vi "IMU_Logger_simple.vi"() -> ()   [LabVIEW 2013]
uses:
  IMU_Data_Type_Def.ctl
  <vilib>/Utility/file.llb/Write To Spreadsheet File (DBL).vi
panel:
  out "Less then 100Hz":bool
  out "IMU_Data_simple":T1
  out "Elapsed Time":u32
  in  "Stop Button":bool
  out "error out":errorcluster
  out "Filename Out":path
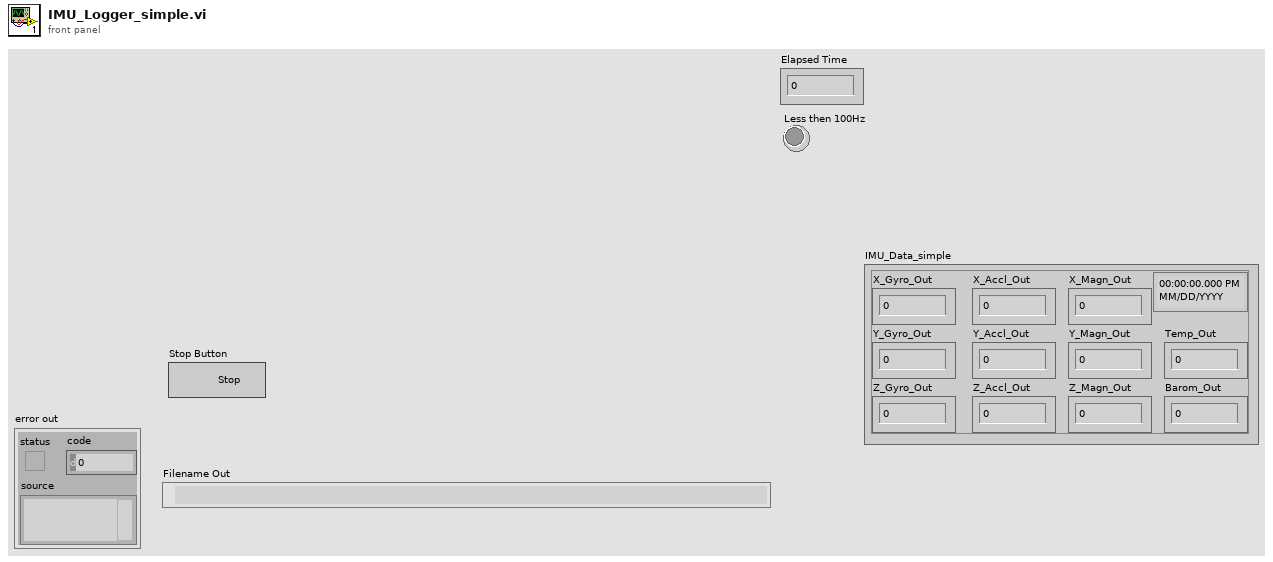
[diagram p1: front panel]
types:
  T1 = typedef "IMU_Data_Type_Def.ctl" = cluster{timestamp, "X_Gyro_Out":dbl, "Y_Gyro_Out":dbl, "Z_Gyro_Out":dbl, "X_Accl_Out":dbl, "Y_Accl_Out":dbl, "Z_Accl_Out":dbl, "X_Magn_Out":dbl, "Y_Magn_Out":dbl, "Z_Magn_Out":dbl, "Temp_Out":dbl, "Barom_Out":dbl}
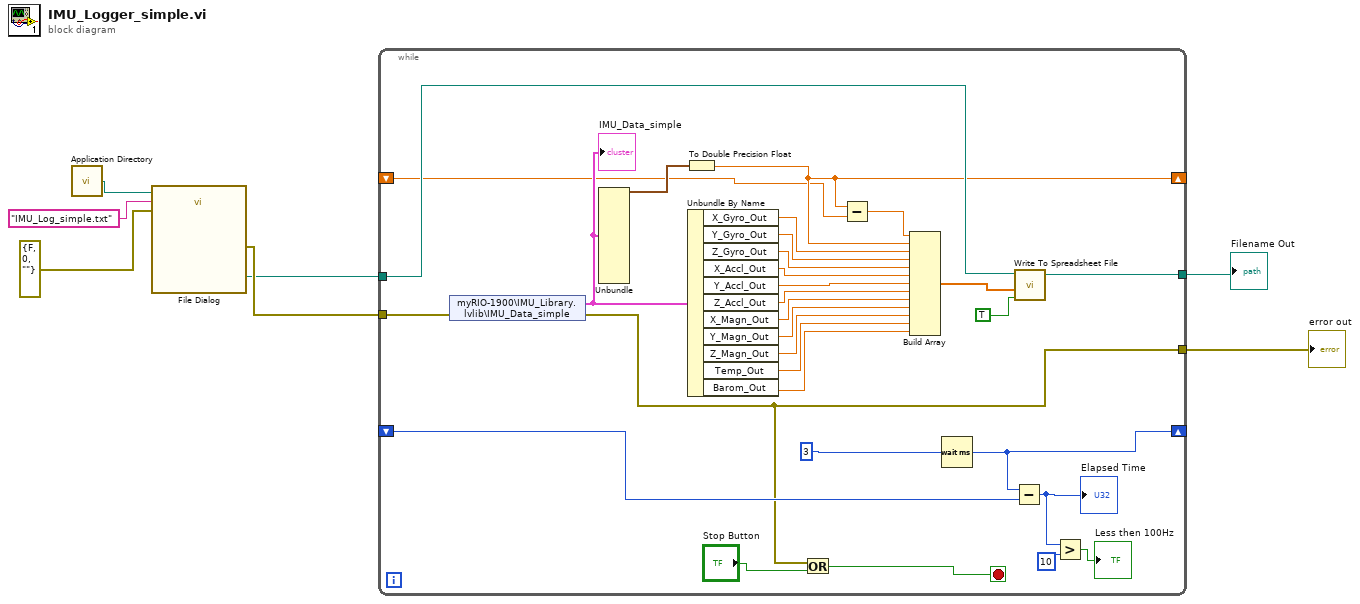
[diagram p0: block diagram]
diagram:
  n1 = call <vilib>:"Application Directory.vi"() -> ("Application Directory"=w7:path)
  n2 = call "File Dialog"("start path"=w7, "default name"="IMU_Log_simple.txt" ("name or relative path"), "error in"=errorcluster {"status"=FALSE, "code"=0, "source"=""} ("error in (no error)")) -> ("selected path"=w2:path, "error out"=w4:errorcluster)  [unwired: 9 in, 2 out]
  n3 = while {
    shift-right: [w15] -> _
    shift-left: _ -> [w35]
    tunnel: w4 -> [w19]
    tunnel: [w18] -> w3
    tunnel: w2 -> [w17]
    tunnel: [w16] -> w1
    shift-right: [w9] -> _
    shift-left: _ -> [w8]
    stop <- w24 stop-if-true
    n4 = shared-variable "myRIO-1900\\IMU_Library.lvlib\\IMU_Data_simple"(error in=w19) -> (w21:T1, error out=w18:errorcluster)
    "IMU_Data_simple" <- w21
    n5 = Unbundle(w21) -> (w20:timestamp)  [unwired: 11 out]
    n6 = To Double Precision Float(number=w20) -> (double precision float=w9:dbl)
    n7 = Unbundle By Name(w21) -> ("X_Gyro_Out"=w34:dbl, "Y_Gyro_Out"=w33:dbl, "Z_Gyro_Out"=w32:dbl, "X_Accl_Out"=w31:dbl, "Y_Accl_Out"=w11:dbl, "Z_Accl_Out"=w30:dbl, "X_Magn_Out"=w29:dbl, "Y_Magn_Out"=w28:dbl, "Z_Magn_Out"=w27:dbl, "Temp_Out"=w26:dbl, "Barom_Out"=w25:dbl)
    n8 = Or(x=w18, y="Stop Button") -> (x .or. y?=w24:bool)
    n9 = Subtract(x=w9, y=w8) -> (x-y=w10:dbl)
    n10 = Build Array(w10, w9, w34, w33, w32, w31, w11, w30, w29, w28, w27, w26, w25) -> (w22:dbl[])
    n11 = Wait (ms)(milliseconds to wait=u32 3) -> (millisecond timer value=w15:u32)
    n12 = Subtract(x=w15, y=w35) -> (x-y=w14:u32)
    "Elapsed Time" <- w14
    n13 = call-poly <vilib>:"Write To Spreadsheet File.vi"("append to file? (new file:F)"=TRUE, "1D data"=w22, "file path (dialog if empty)"=w17) -> ("new file path (Not A Path if cancelled)"=w16:path)  [unwired: 5 in]
    n14 = Greater?(x=w14, y=u32 10) -> (0:→"Less then 100Hz":bool)
  }
  "error out" <- w3
  "Filename Out" <- w1
